vi "Set Configuration.vi"(8 "error in (no error)":errorcluster, 11 "Digital Control in":refnum<class "Digital Control.lvclass">) -> (0 "error out":errorcluster, 3 "Digital Control out":refnum<class "Digital Control.lvclass">)   [LabVIEW 2015, in "Digital Control.lvclass"]
uses:
  Digital Control.lvclass
  IO Class/Type.ctl
  Output Signal/Output Signal.lvclass
  IO Class/IO Class.lvclass
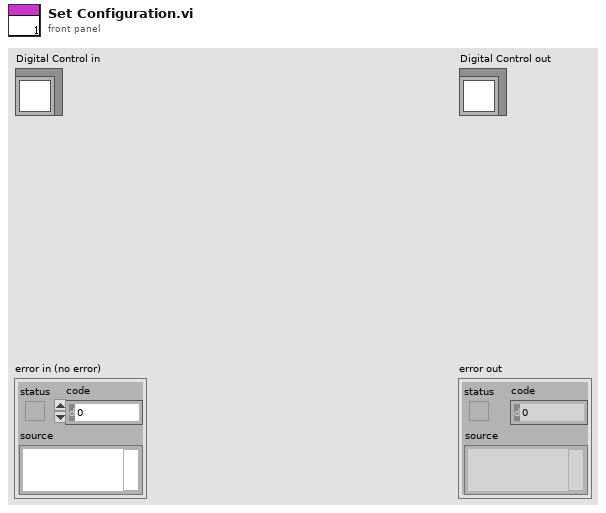
[diagram p1: front panel]
types:
  T1 = typedef "IO Class.lvclass/Type.ctl" = cluster{"Type":string}
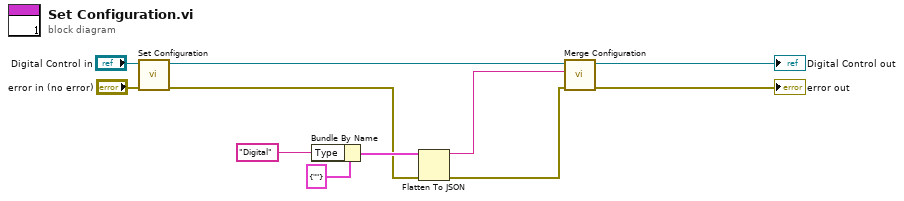
[diagram p0: block diagram]
diagram:
  n1 = call-parent "Set Configuration.vi"("error in (no error)"="error in (no error)", "Output Signal in"="Digital Control in") -> ("error out"=w4:errorcluster, "Output Signal out"=w3:refnum<class "Digital Control.lvclass">)  [unwired: 8 in]
  n2 = Bundle By Name(cluster=T1 {"Type"=""} ("Type"), "Type"="Digital") -> (w8:T1)
  n3 = Flatten To JSON(anything=w8, error in (no error)=w4) -> (JSON string=w6:string, 11:w7:errorcluster)  [unwired: 1 in]
  n4 = call "Merge Configuration.vi"("error in (no error)"=w7, "Additional Configuration"=w6, "IO Class in"=w3) -> ("error out"=→"error out":errorcluster, "IO Class out"=→"Digital Control out":refnum<class "Digital Control.lvclass">)  [unwired: 7 in]
